vi "Infect Test.vi"   [LabVIEW 2017, in "Tests.lvlib"]
uses:
  Tests.lvlib
  Infect Target.vi
  src/Eulogy/Eulogy.lvlib
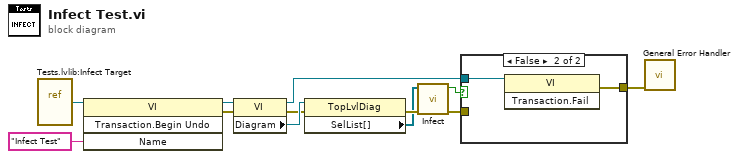
[diagram p0: block diagram]
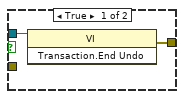
[diagram p2: hidden frame]
diagram:
  n1 = vi-ref "Tests.lvlib:Infect Target.vi"() -> (w7:refnum<vi>)
  n2 = invoke class="VI" method="Transaction.Begin Undo"(reference=w7, "Name"="Infect Test") -> (reference out=w10:refnum<vi>, error out=w8:errorcluster)  [unwired: 2 in, 2 out]
  n3 = property class="VI"(reference=w10, error in=w8) -> (reference out=w1:refnum<vi>, error out=w11:errorcluster, "Diagram"=w12:refnum<vi>)
  n4 = property class="TopLvlDiag"(reference=w12, error in=w11) -> (error out=w5:errorcluster, "SelList[]"=w2:refnum<vi>[])  [unwired: 1 out]
  n5 = call "Infect.vi"("Error In"=w5, "Selection List[]"=w2) -> ("Error Out"=w4:errorcluster, "Change Made?"=w3:bool)  [unwired: 8 in]
  n6 = case shown="False" w3 {
    tunnel: [w14 w16] -> w6
    tunnel: w4 -> [_ _]
    tunnel: w1 -> [w13 w15]
    frame True {
      n7 = invoke class="VI" method="Transaction.End Undo"(reference=w13) -> (error out=w14:errorcluster)  [unwired: 2 in, 2 out]
    }
    frame False {
      n8 = invoke class="VI" method="Transaction.Fail"(reference=w15) -> (error out=w16:errorcluster)  [unwired: 2 in, 2 out]
    }
  }
  n9 = call <vilib>:"General Error Handler.vi"("error in (no error)"=w6) -> ()  [unwired: 10 in, 5 out]
